vi "Write Payload.vi"(7 "Binary (F = Text)":bool, 8 "error in (no error)":errorcluster, 10 "Payload":string, 11 "GodotServer in":refnum<class "GodotServer.lvclass">) -> (0 "error out":errorcluster, 3 "GodotServer out":refnum<class "GodotServer.lvclass">)   [LabVIEW 2020, in "GodotLV.lvlib" / "GodotServer.lvclass"]
doc: "Writes a payload to the WebSocket stream. The format will be dependent on the implementation of the web app.\n\nGodot binary data is Little-Endian."
uses:
  GodotServer.lvclass
  lv-stream/stream/Stream/Stream.lvclass
  lv-stream-websocket/Stream-Websocket/WebsocketStream/WebsocketStream.lvclass
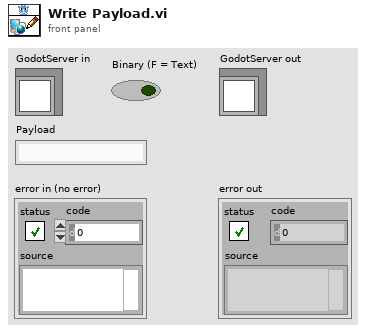
[diagram p1: front panel]
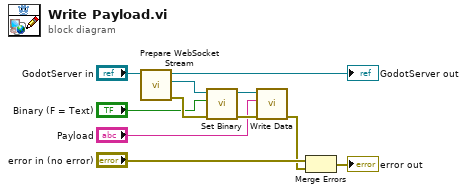
[diagram p0: block diagram]
diagram:
  n1 = call "Prepare WebSocket Stream.vi"("GodotServer in"="GodotServer in") -> ("error out"=w11:errorcluster, "WebsocketStream"=w1:refnum<class "WebsocketStream.lvclass">, "GodotServer out"=→"GodotServer out":refnum<class "GodotServer.lvclass">)  [unwired: 8 in]
  n2 = call "Set Binary.vi"("error in (no error)"=w11, "Binary"="Binary (F = Text)", "WebsocketStream in"=w1) -> ("error out"=w10:errorcluster, "WebsocketStream out"=w4:refnum<class "WebsocketStream.lvclass">)  [unwired: 7 in]
  n3 = call "Write Data.vi"("error in (no error)"=w10, "Data"="Payload", "Stream in"=w4) -> ("error out"=w5:errorcluster)  [unwired: 7 in, 1 out]
  n4 = Merge Errors("error in (no error)", w5) -> (→"error out":errorcluster)
